vi "窗口看门狗实验.vi"   [LabVIEW 2011]
uses:
  <vilib>/STM32_DriverVI_Interface_F4/WDG/WWDG_PSC_F4.ctl
  <vilib>/STM32_DriverVI_Interface_F4/Timer/TIMX Interrupt_F4.ctl
  <vilib>/STM32_DriverVI_Interface_F4/Interrupt/PreemptionPriority_2_F4.ctl
  <vilib>/STM32_DriverVI_Interface_F4/Interrupt/SubPriority_2_F4.ctl
  <vilib>/eio/EIO_TerminalDirection.ctl
  <vilib>/STM32_DriverVI_Interface_F4/GPIO_EIO/GPO_EIO_Inner_F4.vi
  <vilib>/STM32_DriverVI_Interface_F4/Timer/TIM Priority Set_2_F4.vi
  <vilib>/eio/EIONode/EIONode.xnode
types:
  T1 = typedef "SubPriority_2_F4.ctl" = enum8{"Priority_0（High）", "Priority_1", "Priority_2", "Priority_3（Low）"}
  T2 = typedef "PreemptionPriority_2_F4.ctl" = enum8{"Priority_0（Highest）", "Priority_1", "Priority_2", "Priority_3（Lowest）"}
  T3 = typedef "TIMX Interrupt_F4.ctl" = u8
  T4 = typedef "WWDG_PSC_F4.ctl" = u8
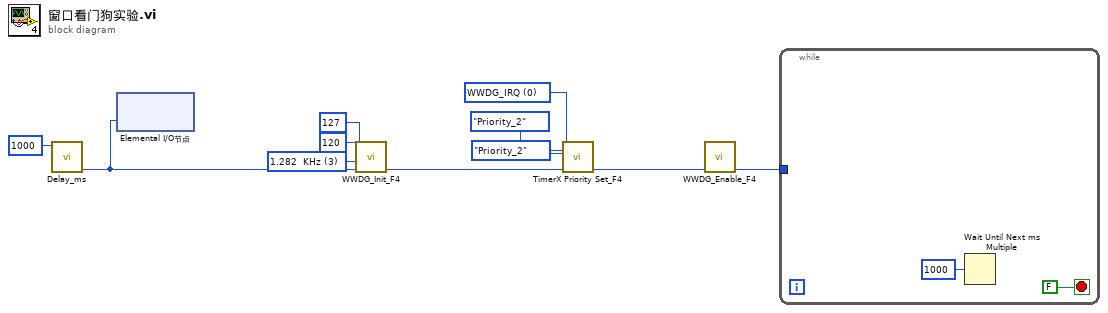
[diagram p0: block diagram]
diagram:
  w5 = T3 0 items=["WWDG_IRQ"=0, "RTC_WKUP_IRQ"=3, "RTC_Alarm_IRQ"=41, "TIM1_BRK_TIM9_IRQ"=24, "TIM1_UP_TIM10_IRQ"=25, "TIM1_TRG_COM_TIM11_IRQ"=26, "TIM1_CC_IRQ"=27, "TIM2_IRQ"=28, "TIM3_IRQ"=29, "TIM4_IRQ"=30, "TIM5_IRQ"=50, "TIM6_IRQ"=54, "TIM7_IRQ"=55, "TIM8_BRK_TIM12_IRQ"=43, "TIM8_UP_TIM13_IRQ"=44, "TIM8_TRG_COM_TIM14_IRQ"=45, "TIM8_CC_IRQ"=46] ("TIM 中断号设置")
  w9 = T4 3 items=["10.25  KHz", "5.127  KHz", "2.563  KHz", "1.282  KHz"] ("WWDG 预分频时基")
  n1 = call <vilib>:"Delay_ms.vi"("time_ms"=u16 1000) -> ("err_out"=w10:u8)  [unwired: 10 in]
  n2 = xnode "Elemental I/O节点"("LED_1"=w10) -> ()  [unwired: 1 in, 1 out]
  n3 = call <vilib>:"WWDG_Init_F4.vi"("err_in"=w10, "WWDG 预分频时基"=w9, "W[6:0] ARR"=u8 120, "T[6:0] ARR"=u8 127) -> ("err_out"=w6:u8)  [unwired: 7 in]
  n4 = call-poly <vilib>:"TimerX Priority Set_F4.vi"("err_in"=w6, "响应优先级"=SubPriority_2_F4."Priority_2", "抢占优先级"=PreemptionPriority_2_F4."Priority_2", "IO 中断号设置"=w5) -> ("err_out"=w2:u8)  [unwired: 6 in, 1 out]
  n5 = call <vilib>:"WWDG_Enable_F4.vi"("err_in"=w2) -> ("err_out"=w1:u8)  [unwired: 10 in]
  n6 = while {
    tunnel: w1 -> [_]
    stop <- FALSE stop-if-true
    n7 = Wait Until Next ms Multiple(millisecond multiple=u32 1000 ("毫秒倍数")) -> ()  [unwired: 1 out]
  }
